vi "LogThrustStringCreator.vi"(1 "rpm":dbl[](array[numeric]), 2 "Tau":dbl[](array[numeric])) -> (0 "output":string)   [LabVIEW 2014]
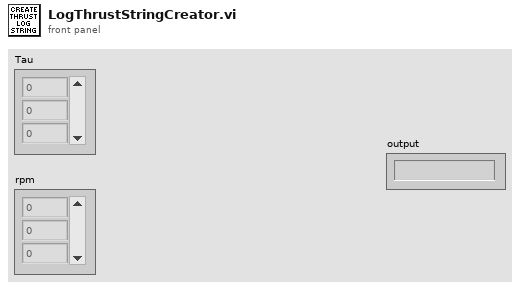
[diagram p1: front panel]
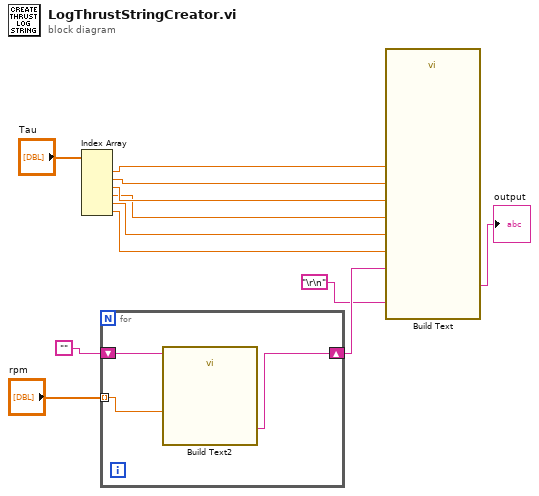
[diagram p0: block diagram]
diagram:
  n1 = Index Array(array="Tau") -> (element #1=w11:dbl, element #2=w10:dbl, element #3=w9:dbl, element #4=w8:dbl, element #5=w7:dbl, element #6=w6:dbl)  [unwired: 6 in]
  n2 = for {
    tunnel: "rpm" -> [w15] mode=indexing
    shift-right: [w14] -> w3
    shift-left: "" -> [w13]
    n3 = call "Build Text2"("Beginning Text"=w13, "value"=w15) -> ("Result"=w14:string)  [unwired: 12 in, 1 out]
  }
  n4 = call "Build Text"("roll"=w8, "yaw"=w6, "EOL"="\r\n", "surge"=w11, "sway"=w10, "heave"=w9, "pitch"=w7, "rpm"=w3) -> ("Result"=→"output":string)  [unwired: 6 in, 1 out]
